vi "PPMS.setAngle.vi"(8 "error in (no error)":errorcluster, 10 "Data":variant, 11 "instrument.PPMS":refnum<class "instrument.PPMS.lvclass">) -> (0 "error out":errorcluster, 3 "instrument.PPMS out":refnum<class "instrument.PPMS.lvclass">)   [LabVIEW 2019, in "instrument.PPMS.lvclass"]
uses:
  instrument.PPMS.lvclass
  <userlib>/LevyLab/Instrument Framework/Instrument Types/Cryostat/Typedefs/setAngle--cluster.ctl
  instrument.PPMS.lvclass/instrument.PPMS.ctl
  4b96368c-9f69-47f8-baf0-4454378acd80.vi
  <vilib>/JDP Science/JSONtext/JSON text to Variant.vi
  <vilib>/JDP Science/JSONtext/LVClass Serializer/JSONtext LVClass Serializer.lvclass
  <userlib>/LevyLab/Instrument Framework/Instrument Types/Cryostat/Instrument.Cryostat.lvclass
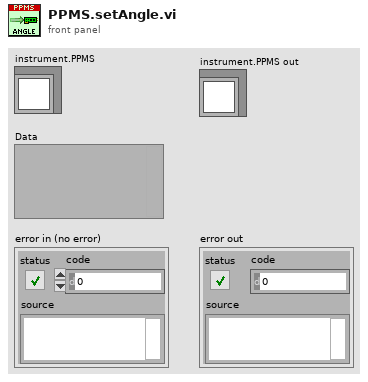
[diagram p1: front panel]
types:
  T1 = typedef "Instrument.Cryostat.lvclass/setAngle--cluster.ctl" = cluster{"angle":dbl, "rate":dbl, "channel":i32}
  T2 = enum16{"0", "1", "2", "3", "4", "5", "6", "7", "8", "9", "10", "11", "12", "13", "14"}
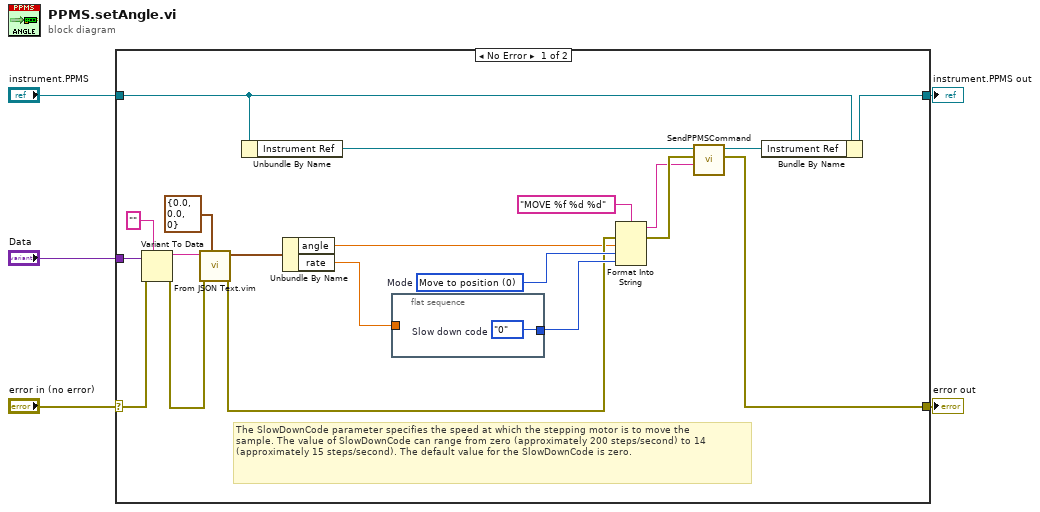
[diagram p0: block diagram]
diagram:
  n1 = case shown="No Error" "error in (no error)" {
    selector: "error in (no error)" -> [w14 w28]
    tunnel: "Data" -> [w15 _]
    tunnel: [w24 w28] -> w4
    tunnel: "instrument.PPMS" -> [w6 w27]
    tunnel: [w7 w27] -> w1
    frame No Error {
      w22 = u16 0 items=["Move to position", "Move to limit", "Redefine current position", ""]  # Mode
      # "The SlowDownCode parameter specifies the speed at which the stepping motor is to move the\nsample. The value of SlowDownCode can range from zero (approximately 200 steps/second) to 14\n(approximately 15 steps/second). The default value for the SlowDownCode is zero."
      n2 = Variant To Data(error in=w14, type="", Variant=w15) -> (data=w17:string, error out=w13:errorcluster)
      n3 = call "From JSON Text.vim"("Data Type and Default Value"=T1 {"angle"=0.0, "rate"=0.0, "channel"=0} ("Set Angle"), "error in (no error)"=w13, "JSON"=w17) -> ("error out"=w12:errorcluster, "Data out"=w16:T1)  [unwired: 7 in]
      n4 = Unbundle By Name(w6) -> ("Instrument Ref"=w25:refnum<k24>)
      n5 = Unbundle By Name(w16) -> ("angle"=w10:dbl, "rate"=w9:dbl)
      n6 = flat-sequence {
        tunnel: [w26] -> w19
        tunnel: w9 -> [_]
        frame #0 {
          w26 = T2."0"  # Slow down code
        }
      }
      n7 = Format Into String(format string="MOVE %f %d %d", error in=w12, w10, w22, w19) -> (resulting string=w20:string, error out=w21:errorcluster)  [unwired: 1 in]
      n8 = call "SendPPMSCommand.vi"("PpmsCommand"=w20, "error in (no error)"=w21, "Instrument Ref In"=w25) -> ("error out"=w24:errorcluster, "Instrument Ref Out"=w8:refnum<k24>)  [unwired: 4 in, 3 out]
      n9 = Bundle By Name(cluster=w6, "Instrument Ref"=w8) -> (w7:refnum<class "instrument.PPMS.lvclass">)
    }
    frame Error {
    }
  }
  "error out" <- w4
  "instrument.PPMS out" <- w1
